vi "Single Pulse Generator .vi"() -> ()   [LabVIEW 2019, in "Part of Main VIs.lvlib" / "Tachometer Library.lvlib"]
uses:
  <vilib>/Platform/TimedLoop/XDataNode/timing_clust.ctl
  <vilib>/Platform/TimedLoop/XDataNode/nitl_modes.ctl
  <vilib>/Platform/TimedLoop/XDataNode/wakeup.ctl
  <vilib>/DAQmx/create/channels.llb/DAQmx Create Channel (CO-Pulse Generation-Time).vi
  <vilib>/DAQmx/configure/timing.llb/DAQmx Timing (Implicit).vi
  <vilib>/Platform/TimedLoop/XDataNode/XDataNode.xnode
  Tachometer Library.lvlib
  <resource>/objmgr/daqmx.rc
  <vilib>/Platform/TimedLoop/XDataNode/XDNodeRunTimeDep.lvlib
panel:
  in  "Angular Velocity 2":dbl max=131.94689 format="%#_9g"
  out "Ø Sweep Chart 2":dbl(graph)
  out "Ø(n) 2":dbl
  out "2pi/18 2":dbl
  out "Ø(n-1) 2":dbl
  out "^Ø 2":dbl
  out "Numeric":i32
  out "Iteration of Part of Telemetry 3":i32
  out "^Ø":dbl
  out "Ø(n-1)":dbl
  out "2pi/18":dbl
  out "Ø(n)":dbl
  out "Iteration of Part of Telemetry":i32
  out "Ø Sweep Chart":dbl(graph)
  in  "Angular Velocity":dbl max=131.94689 format="%#_9g"
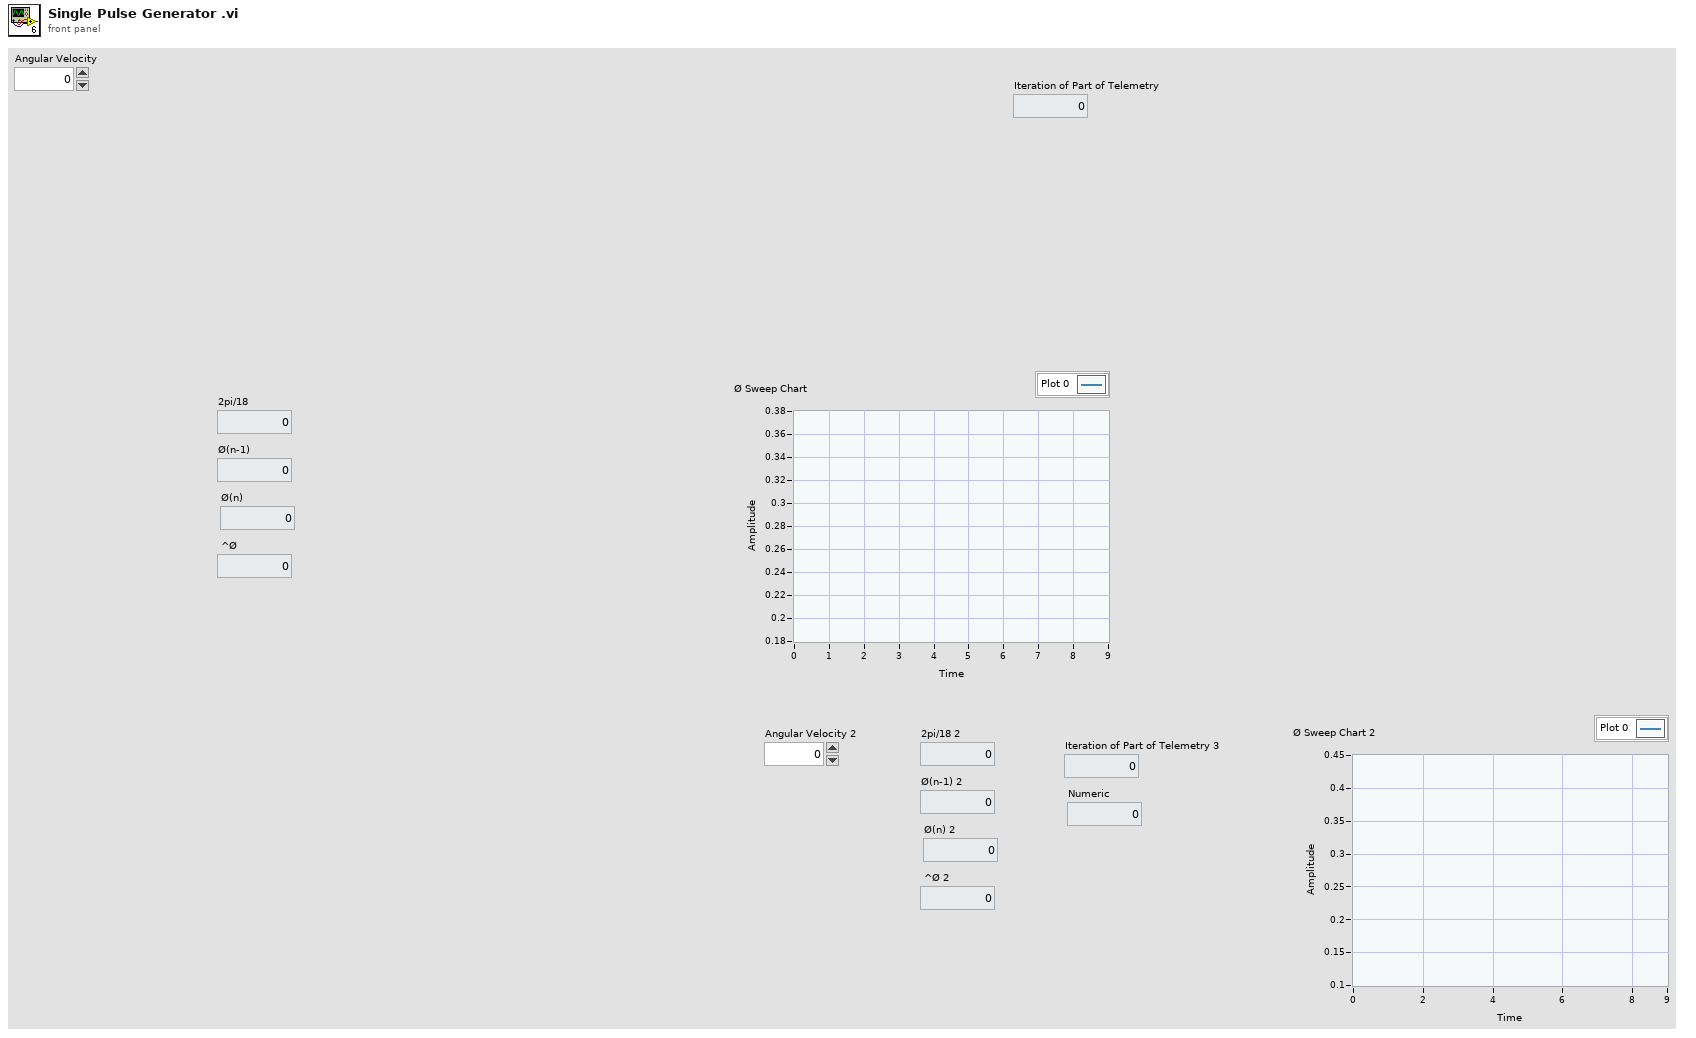
[diagram p1: front panel]
types:
  T1 = typedef "XDNodeRunTimeDep.lvlib/timing_clust.ctl" = cluster{"Expected End [f-1]":u64, "Actual End [f-1]":u64, "Finished Late? [f-1]":bool, "Expected End [i-1]":u64, "Actual End [i-1]":u64, "Finished Late? [i-1]":bool, "Expected Start [i]":u64, "Actual Start [i]":u64, "Expected Start [f]":u64, "Actual Start [f]":u64, "Source Name":string, "Structure Name":string, "Period":i64, "Deadline":i64, "Offset":i64, "Start":i64, "Priority":i32, "Timeout":i32, "Mode":T2, "Wakeup Reason":T3, "Error":errorcluster, "Source Type":string, "Secondary Source Type":string, "Global End Time":u64, "Global Start Time":u64, "Frame Duration":u64, "Iteration Duration":u64, "Assigned CPU":i32, "I/O Scan Engine Mode":u32}
  T2 = typedef "XDNodeRunTimeDep.lvlib/nitl_modes.ctl" = enum32{"No Change", "Process missed periods, maintain original phase", "Discard missed periods, maintain original phase", "Process missed periods, ignore original phase", "Discard missed periods, ignore original phase"}
  T3 = typedef "XDNodeRunTimeDep.lvlib/wakeup.ctl" = enum32{"Normal", "Aborted", "Asynchronous wakeup", "Timing source error", "Timed loop error", "Timeout"}
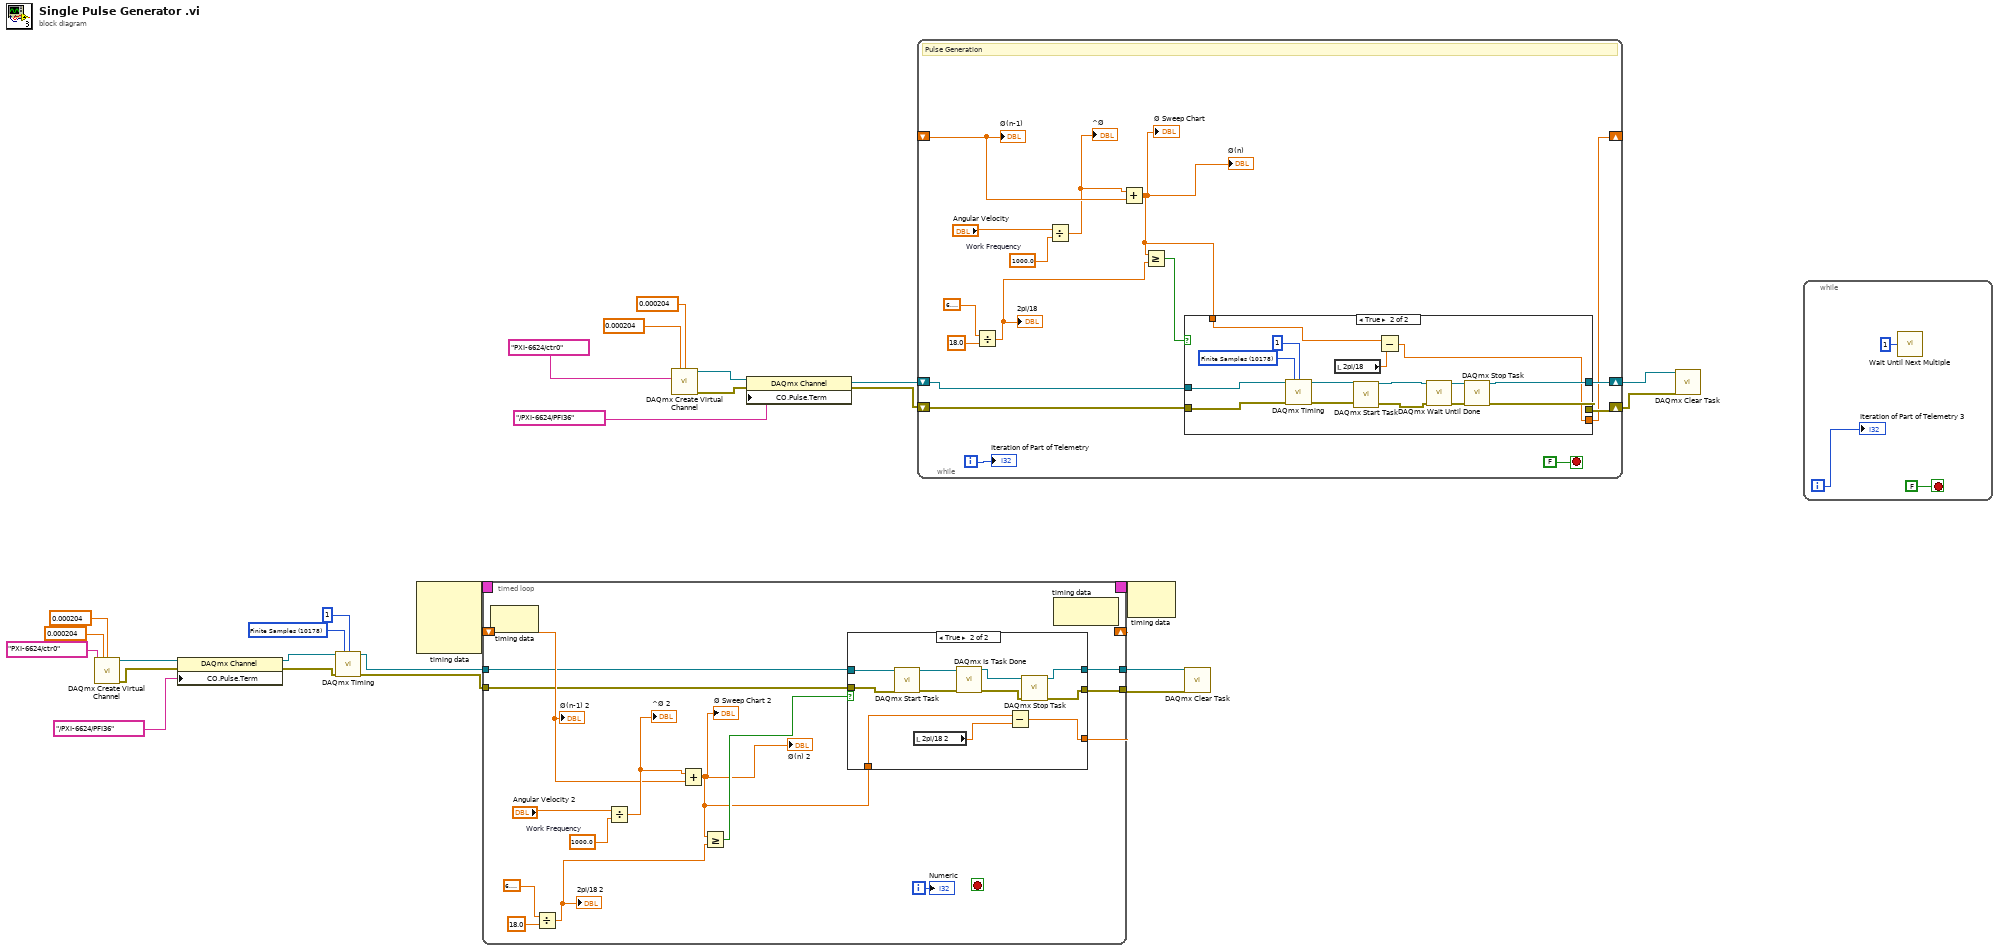
[diagram p0: block diagram]
diagram:
  w17 = 10178 items=["Finite Samples"=10178, "Continuous Samples"=10123, "Hardware Timed Single Point"=12522] ("sample mode")
  n1 = call-poly <vilib>:"DAQmx Create Virtual Channel.vi"("high time"=0.000204, "low time"=0.000204, "counter"=tag "PXI-6624/ctr0") -> ("task out"=w26:refnum<k21>, "error out"=w25:errorcluster)  [unwired: 11 in]
  n2 = property class="DAQmx Channel"(reference=w26, error in=w25, "CO.Pulse.Term"=tag "/PXI-6624/PFI36") -> (reference out=w15:refnum<k21>, error out=w16:errorcluster)
  n3 = call-poly <vilib>:"DAQmx Timing.vi"("task/channels in"=w15, "sample mode"=w17, "samples per channel"=1, "error in"=w16) -> ("task out"=w14:refnum<k21>, "error out"=w13:errorcluster)  [unwired: 10 in]
  n4 = node-c288() -> (w20:T1)  [unwired: 4 in]
  n5 = timed-loop {
    tunnel: [w40] -> w11
    shift-right: [w29] -> _
    shift-left: _ -> [w31]
    timing: w20 -> [_]
    timing-out: [_] -> w19
    tunnel: w13 -> [w27]
    tunnel: w14 -> [w28]
    tunnel: [w41] -> w12
    i -> [w39]
    stop <- _ stop-if-true
    w35 = 1000.0  # Work Frequency
    n6 = node-c288() -> ()  [unwired: 1 in, 1 out]
    n7 = Divide(x=6.283185307179586, y=18.0) -> (x/y=w38:dbl)
    "2pi/18 2" <- w38
    n8 = Divide(x="Angular Velocity 2", y=w35) -> (x/y=w34:dbl)
    "^Ø 2" <- w34
    n9 = Add(x=w34, y=w31) -> (x+y=w30:dbl)
    "Ø(n) 2" <- w30
    "Ø Sweep Chart 2" <- w30
    n10 = Greater Or Equal?(x=w30, y=w38) -> (x >= y?=w32:bool)
    n11 = case shown="True" w32 {
      tunnel: [_ w46] -> w41
      tunnel: [_ w45] -> w40
      tunnel: w30 -> [w44 w54]
      tunnel: [w44 w53] -> w29
      tunnel: w28 -> [_ w50]
      tunnel: w27 -> [_ w49]
      frame False {
      }
      frame True {
        n12 = call <vilib>:"DAQmx Start Task.vi"("task/channels in"=w50, "error in"=w49) -> ("task out"=w52:refnum<k21>, "error out"=w51:errorcluster)  [unwired: 12 in]
        n13 = local read "2pi/18 2"() -> (w55:dbl)
        n14 = call <vilib>:"DAQmx Is Task Done.vi"("task/channels in"=w52, "error in"=w51) -> ("task out"=w48:refnum<k21>, "error out"=w47:errorcluster)  [unwired: 11 in, 1 out]
        n15 = Subtract(x=w54, y=w55) -> (x-y=w53:dbl)
        n16 = call <vilib>:"DAQmx Stop Task.vi"("task/channels in"=w48, "error in"=w47) -> ("task out"=w46:refnum<k21>, "error out"=w45:errorcluster)  [unwired: 12 in]
      }
    }
    n17 = node-c288() -> ()  [unwired: 1 in, 1 out]
    "Numeric" <- w39
    "Ø(n-1) 2" <- w31
  }
  n18 = call-poly <vilib>:"DAQmx Create Virtual Channel.vi"("high time"=0.000204 ("y"), "low time"=0.000204, "counter"=tag "PXI-6624/ctr0") -> ("task out"=w8:refnum<k21>, "error out"=w7:errorcluster)  [unwired: 11 in]
  n19 = property class="DAQmx Channel"(reference=w8, error in=w7, "CO.Pulse.Term"=tag "/PXI-6624/PFI36") -> (reference out=w4:refnum<k21>, error out=w6:errorcluster)
  n20 = while {
    shift-right: [w56] -> _
    shift-left: _ -> [w65]
    shift-right: [w63] -> w5
    shift-left: w4 -> [w58]
    shift-right: [w62] -> w1
    shift-left: w6 -> [w61]
    i -> [w66]
    stop <- FALSE stop-if-true
    w67 = 1000.0  # Work Frequency
    # "Pulse Generation"
    n21 = Divide(x=6.283185307179586, y=18.0) -> (x/y=w70:dbl)
    "2pi/18" <- w70
    n22 = Divide(x="Angular Velocity", y=w67) -> (x/y=w60:dbl)
    "^Ø" <- w60
    n23 = Add(x=w60, y=w65) -> (x+y=w59:dbl)
    "Ø(n)" <- w59
    "Ø Sweep Chart" <- w59
    n24 = Greater Or Equal?(x=w59, y=w70) -> (x >= y?=w64:bool)
    n25 = case shown="True" w64 {
      tunnel: [w72 w75] -> w56
      tunnel: [w74 w81] -> w63
      tunnel: [w73 w80] -> w62
      tunnel: w58 -> [w74 w79]
      tunnel: w61 -> [w73 w78]
      tunnel: w59 -> [w72 w77]
      frame False {
      }
      frame True {
        w89 = 10178 items=["Finite Samples"=10178, "Continuous Samples"=10123, "Hardware Timed Single Point"=12522] ("sample mode")
        n26 = call-poly <vilib>:"DAQmx Timing.vi"("task/channels in"=w79, "sample mode"=w89, "samples per channel"=1, "error in"=w78) -> ("task out"=w87:refnum<k21>, "error out"=w86:errorcluster)  [unwired: 10 in]
        n27 = local read "2pi/18"() -> (w76:dbl)
        n28 = call <vilib>:"DAQmx Start Task.vi"("task/channels in"=w87, "error in"=w86) -> ("task out"=w83:refnum<k21>, "error out"=w82:errorcluster)  [unwired: 12 in]
        n29 = Subtract(x=w77, y=w76) -> (x-y=w75:dbl)
        n30 = call <vilib>:"DAQmx Wait Until Done.vi"("task/channels in"=w83, "error in"=w82) -> ("task out"=w85:refnum<k21>, "error out"=w84:errorcluster)  [unwired: 12 in]
        n31 = call <vilib>:"DAQmx Stop Task.vi"("task/channels in"=w85, "error in"=w84) -> ("task out"=w81:refnum<k21>, "error out"=w80:errorcluster)  [unwired: 12 in]
      }
    }
    "Ø(n-1)" <- w65
    "Iteration of Part of Telemetry" <- w66
  }
  n32 = node-c288(w19) -> ()  [unwired: 1 out]
  n33 = call <vilib>:"DAQmx Clear Task.vi"("task in"=w12, "error in"=w11) -> ()  [unwired: 13 in, 1 out]
  n34 = call <vilib>:"DAQmx Clear Task.vi"("task in"=w5, "error in"=w1) -> ()  [unwired: 13 in, 1 out]
  n35 = while {
    i -> [w90]
    stop <- FALSE stop-if-true
    n36 = call "Wait Until Next Multiple"("Count(mSec)"=u32 1) -> ()  [unwired: 1 out]
    "Iteration of Part of Telemetry 3" <- w90
  }
